vi "ArmSetPositionDemands.vi"(9 "SetExtendPositonDemand(in)":dbl, 10 "SetLIftPostionDemand(d)":dbl, 11 "SetRotatePostionDemand(d)":dbl) -> ()   [LabVIEW 2020]
doc: "Setters for Arm\nInputs:\n--SetRotatePositionDemand(d)--\n--SetLiftPostionDemand(d)--\n--SetExtendPostionDemand(in)--"
uses:
  ArmGlobal.vi
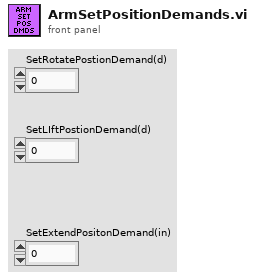
[diagram p1: front panel]
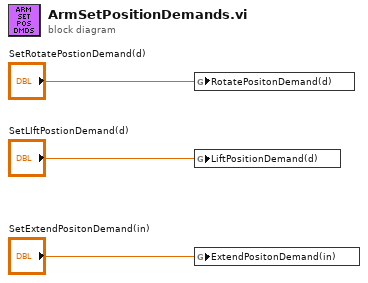
[diagram p0: block diagram]
diagram:
  n1 = global write "ArmGlobal.vi" "RotatePositonDemand(d)"("SetRotatePostionDemand(d)") -> ()
  n2 = global write "ArmGlobal.vi" "LiftPositionDemand(d)"("SetLIftPostionDemand(d)") -> ()
  n3 = global write "ArmGlobal.vi" "ExtendPositonDemand(in)"("SetExtendPositonDemand(in)") -> ()
